vi "RtkNemaStats.vi"(11 "Element":string) -> (0 "GPS Type":string, 1 "Numeric Time Stamp":dbl, 2 "IP-Port":string, 3 "Array of Nema Parts":string[](array[string]), 4 "RTK = T":bool)   [LabVIEW 2012]
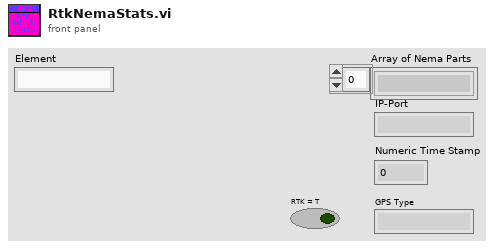
[diagram p1: front panel]
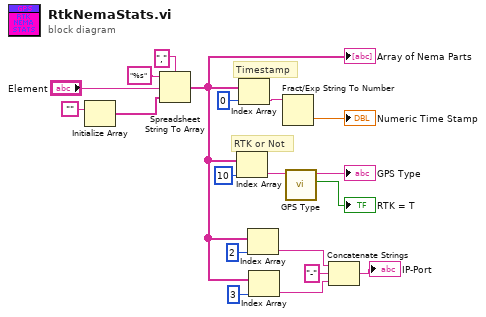
[diagram p0: block diagram]
diagram:
  # "RTK or Not"
  # "Timestamp"
  n1 = Initialize Array("") -> (w12:string[])  [unwired: 1 in]
  n2 = Spreadsheet String To Array(delimiter (Tab)="," ("regular expression"), format string="%s", spreadsheet string="Element", array type (2D Dbl)=w12) -> (array=w5:string[])
  "Array of Nema Parts" <- w5
  n3 = Index Array(array=w5, index=10) -> (element=w18:string)
  n4 = Index Array(array=w5, index=0) -> (element=w15:string)
  n5 = Index Array(array=w5, index=2) -> (element=w3:string)
  n6 = Index Array(array=w5, index=3) -> (element=w2:string)
  n7 = Fract/Exp String To Number(string=w15) -> (number=→"Numeric Time Stamp":dbl)  [unwired: 3 in, 1 out]
  n8 = call "GPS Type.vi"("Nema Def"=w18) -> ("RTK = T"=→"RTK = T":bool, "GPS Type"=→"GPS Type":string)  [unwired: 9 in]
  n9 = Concatenate Strings(w3, "-" ("string"), w2) -> (→"IP-Port":string)
